vi "SV Software Triggering (Analog Edge).vi"(0 "input signals":waveform(dbl)[](array[waveform]), 1 "restart (F = first call)":bool, 2 "force trigger (F)":bool, 5 "level trigger configuration":T1={"level"=0.0, "slope"=1, "hysteresis"=0.0} {"hysteresis" format="%.2p"; "slope" items=["Falling", "Rising"]; "level" format="%.2p"}, 7 "trigger channel index (0)":i32, 9 "mode (FIFO)":enum16{"First In, First Out", "Last Available"}(ring), 11 "error in (no error)":errorcluster, 12 "pretrigger samples (0)":i32) -> (3 "data timestamp":timestamp, 4 "triggered signals":waveform(dbl)[](array[waveform]), 6 "output ready":bool, 8 "new trigger detected":bool, 15 "error out":errorcluster)   [LabVIEW 2017]
doc: "Implements a software trigger. When the trigger is detected on the trigger channel, all signals are triggered so that the channels stay aligned in time. This function requires that each waveform in <B>input signals</B> has equal <B>dt</B> and <B>Y</B> (length). Returns one triggered set of data per call."
uses:
  <vilib>/addons/_NISVFA/_Shared subVIs/Controls/svc_Analog Level Trigger Configuration.ctl
  <vilib>/addons/_NISVFA/_Shared subVIs/Common/svc_Get Array Subset (Index).vi
  <vilib>/addons/_NISVFA/_Shared subVIs/Common/svc_Check for Waveform Parameter Continuity (no state).vi
  <vilib>/addons/_NISVFA/_Shared subVIs/Common/svc_Coerce Index and Length.vi
  <vilib>/addons/_NISVFA/_Shared subVIs/Common/svc_Get SV Channel Info.vi
  <vilib>/measure/mamon.llb/Trigger Detection for 1 Channel.vi
  <vilib>/addons/_NISVFA/_Shared subVIs/Common/svc_Engineering Units to Unit Label.vi
  <vilib>/addons/_NISVFA/_Shared subVIs/Common/svc_Unit Label to Engineering Units.vi
  <vilib>/measure/NI_MAPro.lvlib
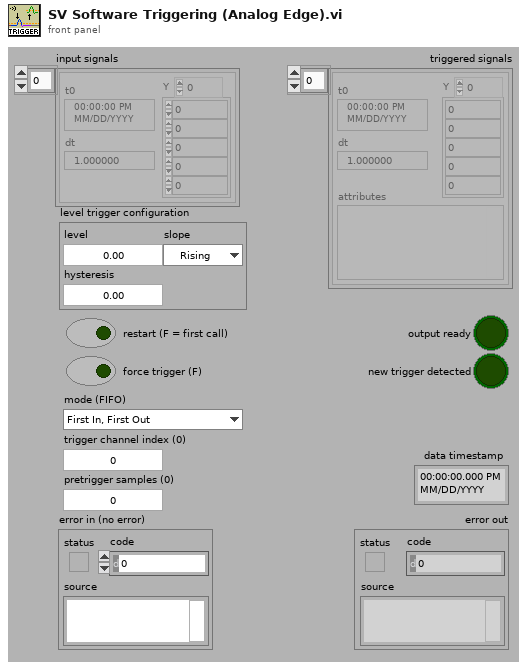
[diagram p1: front panel]
types:
  T1 = typedef "svc_Analog Level Trigger Configuration.ctl" = cluster{"level":dbl, "slope":u16, "hysteresis":dbl}
  T2 = cluster{"dt equal":bool, "array length equal":bool, "number channels change":bool}
  T3 = cluster{"dt":bool, "t0 continuity":bool, "array length":bool, "channel info":bool, "name":bool}
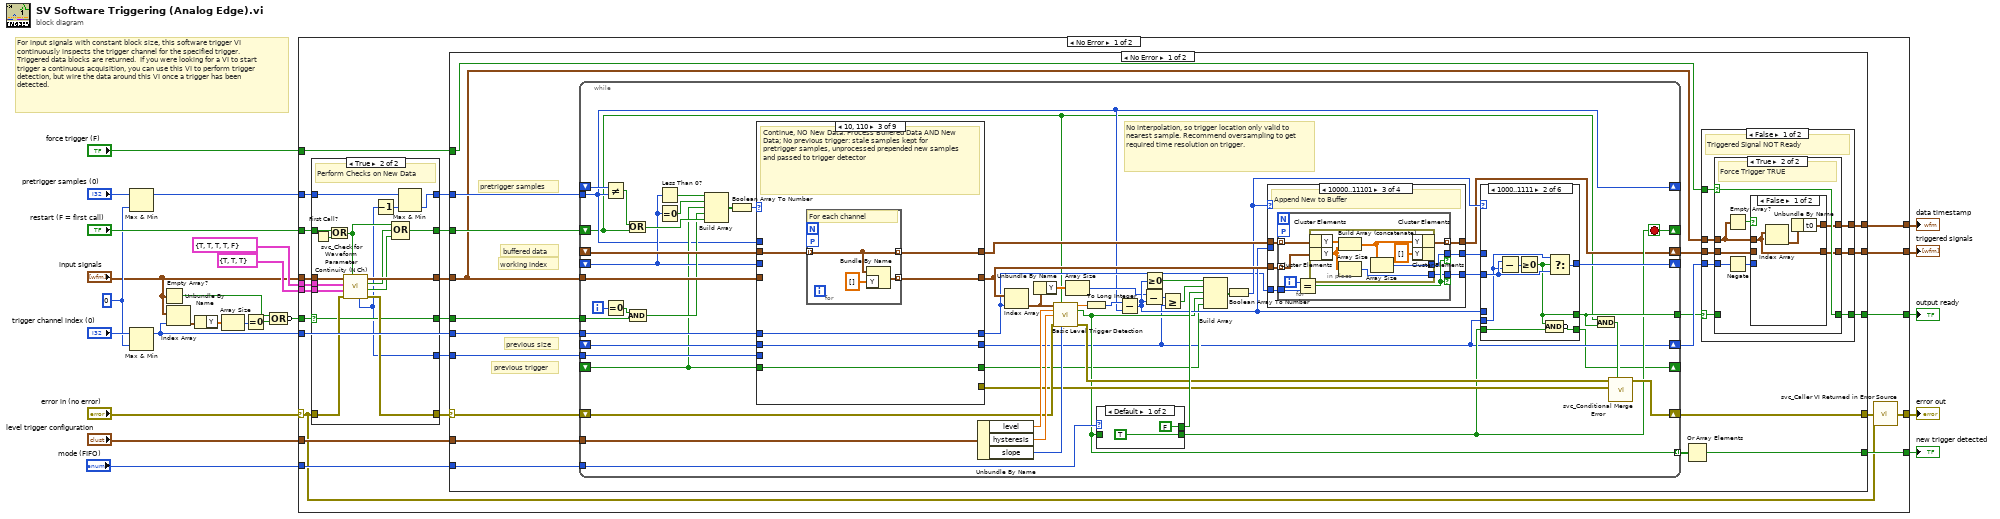
[diagram p0: block diagram]
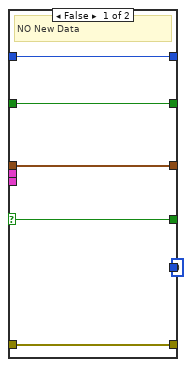
[diagram p2: hidden frame]
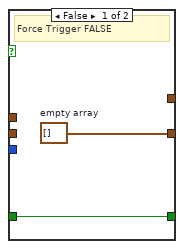
[diagram p3: hidden frame]
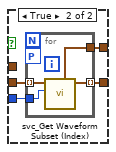
[diagram p4: hidden frame]
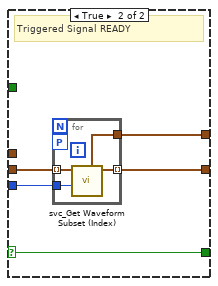
[diagram p5: hidden frame]
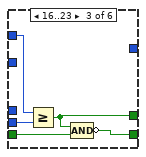
[diagram p7: hidden frame]
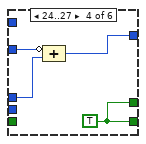
[diagram p8: hidden frame]
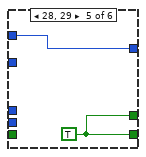
[diagram p9: hidden frame]
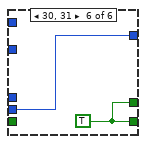
[diagram p10: hidden frame]
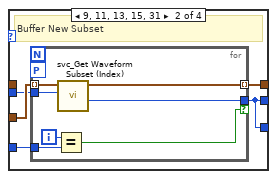
[diagram p12: hidden frame]
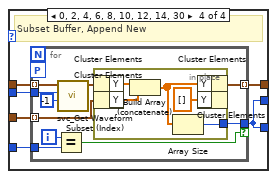
[diagram p13: hidden frame]
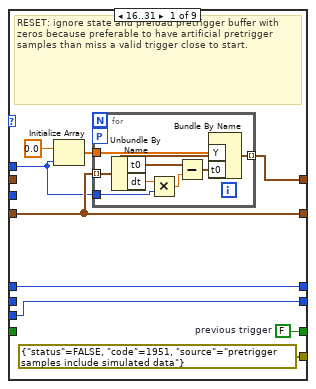
[diagram p14: hidden frame]
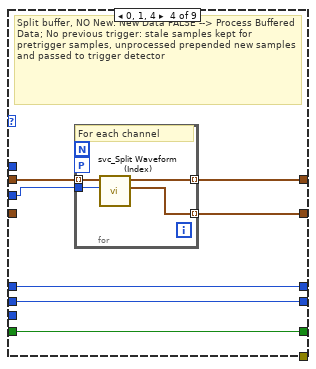
[diagram p16: hidden frame]
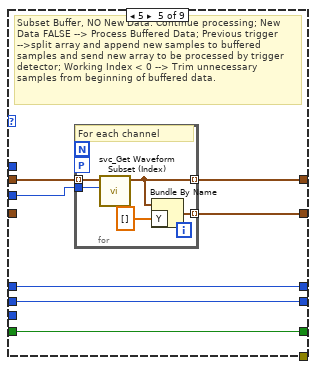
[diagram p17: hidden frame]
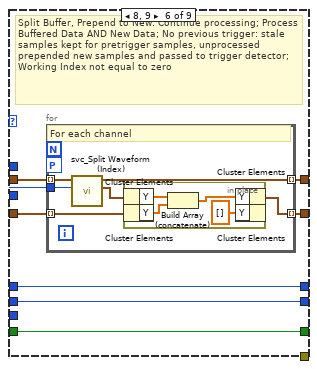
[diagram p18: hidden frame]
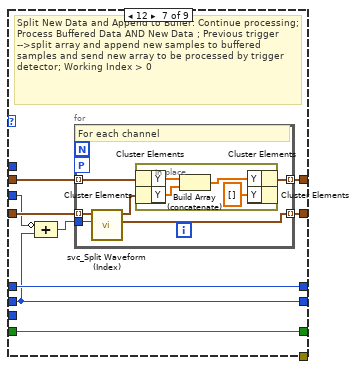
[diagram p19: hidden frame]
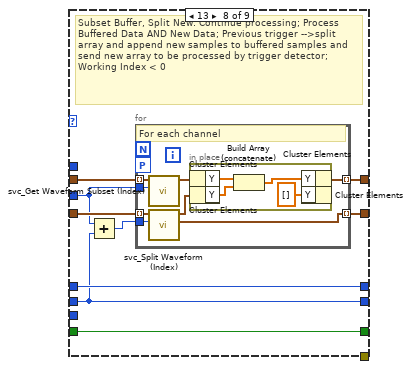
[diagram p20: hidden frame]
diagram:
  w11 = 0 ("y")
  # "For input signals with constant block size, this software trigger VI continuously inspects the trigger channel for the specified trigger. Triggered data blocks are returned.  If you were looking for a VI to start trigger a continuous acquisition, you can use this VI to perform trigger detection, but wire the data around this VI once a trigger has been detected."
  n1 = Max & Min(x="pretrigger samples (0)", y=w11) -> (max(x,y)=w6:i32)  [unwired: 1 out]
  n2 = Max & Min(x="trigger channel index (0)", y=w11) -> (max(x,y)=w13:i32)  [unwired: 1 out]
  n3 = Empty Array?(array="input signals") -> (empty?=w18:bool)
  n4 = Index Array(array="input signals", index=w13) -> (element=w9:waveform(dbl))
  n5 = Unbundle By Name(w9) -> ("Y"=w10:dbl[])
  n6 = Array Size(array=w10) -> (size(s)=w8:i32)
  n7 = Equal To 0?(x=w8) -> (x = 0?=w17:bool)
  n8 = Compound Arithmetic op=OR(w18, w17) -> (invert w4:bool)
  n9 = case shown="No Error" "error in (no error)" {
    selector: "error in (no error)" -> [w26 w380]
    tunnel: "input signals" -> [w42 _]
    tunnel: w13 -> [w47 _]
    tunnel: [w46 _] -> w24
    tunnel: [w45 _] -> w23
    tunnel: [w37 _] -> w22
    tunnel: "level trigger configuration" -> [w44 _]
    tunnel: [w28 w380] -> w20
    tunnel: "restart (F = first call)" -> [w43 _]
    tunnel: T2 {"dt equal"=TRUE, "array length equal"=TRUE, "number channels change"=TRUE} ("checks for multichannel parameters") -> [w40 _]
    tunnel: T3 {"dt"=TRUE, "t0 continuity"=TRUE, "array length"=TRUE, "channel info"=TRUE, "name"=FALSE} ("checks for channel parameter change") -> [w39 _]
    tunnel: "force trigger (F)" -> [w35 _]
    tunnel: w6 -> [w34 _]
    tunnel: w4 -> [w32 _]
    tunnel: "mode (FIFO)" -> [w29 _]
    tunnel: [w25 _] -> w1
    frame No Error {
      n10 = case shown="True" w32 {
        selector: w32 -> [w48 w55]
        tunnel: w43 -> [w50 w70]
        tunnel: w42 -> [w53 w68]
        tunnel: [w53 w67] -> w41
        tunnel: w26 -> [w52 w66]
        tunnel: w40 -> [_ w65]
        tunnel: w39 -> [_ w64]
        tunnel: [w50 w60] -> w38
        tunnel: [w52 w59] -> w36
        tunnel: w34 -> [w51 w57]
        tunnel: [w51 w56] -> w33
        tunnel: [0 ("array length") w54] -> w31
        tunnel: [w48 w55] -> w30
        frame False {
          # "NO New Data"
        }
        frame True {
          # "Perform Checks on New Data"
          n11 = First Call?() -> (First Call?: T/F=w69:bool)
          n12 = Or(x=w70, y=w69) -> (x .or. y?=w61:bool)
          n13 = call <vilib>:"svc_Check for Waveform Parameter Continuity (N Ch).vi"("restart averaging (F)"=w61, "error in (no error)"=w66, "checks for multichannel parameters"=w65, "checks for channel parameter change"=w64, "scaled signal(s)"=w68) -> ("error out"=w59:errorcluster, "multichannel parameter changed"=w62:bool, "waveform parameter changed"=w63:bool, "dup scaled signal(s)"=w67:waveform(dbl)[], "array length"=w54:i32)  [unwired: 2 out]
          n14 = Decrement(x=w54) -> (x-1=w58:i32)
          n15 = Compound Arithmetic op=OR(w61, w63, w62) -> (w60:bool)
          n16 = Max & Min(x=w57, y=w58) -> (min(x,y)=w56:i32)  [unwired: 1 out]
        }
      }
      n17 = case shown="No Error" w36 {
        selector: w36 -> [w84 w379]
        tunnel: w33 -> [w89 _]
        tunnel: w47 -> [w88 _]
        tunnel: [w76 _] -> w46
        tunnel: [w73 _] -> w45
        tunnel: w44 -> [w87 _]
        tunnel: [w72 w379] -> w27
        tunnel: w31 -> [w86 _]
        tunnel: w41 -> [w77 _]
        tunnel: w38 -> [w85 _]
        tunnel: [w81 _] -> w37
        tunnel: w35 -> [w78 _]
        tunnel: w30 -> [w75 _]
        tunnel: w29 -> [w74 _]
        tunnel: [w71 _] -> w25
        frame No Error {
          # "pretrigger samples"
          # "previous size"
          # "previous trigger"
          # "working index"
          # "buffered data"
          n18 = while {
            shift-right: [w131] -> w83
            shift-left: _ -> [w162]
            tunnel: w77 -> [w161]
            shift-right: [w128] -> _
            shift-left: _ -> [w136]
            tunnel: w89 -> [w130]
            tunnel: w88 -> [w160]
            tunnel: [w142] -> w80
            shift-right: [w132] -> w82
            shift-left: _ -> [w159]
            tunnel: w87 -> [w180]
            tunnel: w86 -> [w158]
            shift-right: [w146] -> w72
            shift-left: w84 -> [w179]
            shift-right: [w143] -> _
            shift-left: _ -> [w156]
            tunnel: [w137] -> w79 mode=indexing
            shift-right: [w130] -> _
            shift-left: _ -> [w178]
            tunnel: w75 -> [w173]
            tunnel: w74 -> [w155]
            shift-right: [w135] -> _
            shift-left: w85 -> [w129]
            i -> [w175]
            stop <- w135 stop-if-true
            # "No interpolation, so trigger location only valid to nearest sample. Recommend oversampling to get required time resolution on trigger."
            n19 = Not Equal?(x=w178, y=w130) -> (x != y?=w177:bool)
            n20 = Equal To 0?(x=w175) -> (x = 0?=w174:bool)
            n21 = Or(x=w177, y=w129) -> (x .or. y?=w167:bool)
            n22 = And(x=w174, y=w173) -> (x .and. y?=w157:bool)
            n23 = Less Than 0?(x=w156) -> (x < 0?=w165:bool)
            n24 = Equal To 0?(x=w156) -> (x = 0?=w166:bool)
            n25 = Build Array(w165, w166, w136, w157, w167) -> (w164:bool[])
            n26 = Boolean Array To Number(Boolean array=w164) -> (number=w163:u32)
            n27 = case shown="10, 110" w163 {
              tunnel: w161 -> [w261 w278 _ _ _ w315 w334 w354 w372]
              tunnel: w160 -> [w265 w276 w283 w293 w304 w317 w337 w356 w370]
              tunnel: [w260 w275 w284 w294 w305 w318 w330 w349 w373] -> w132
              tunnel: w162 -> [_ w277 w282 w292 w303 w316 w335 w353 w371]
              tunnel: [w261 w278 w281 w291 w302 w314 w332 w351 w372] -> w147
              tunnel: w159 -> [_ w275 w284 w294 w305 w318 w330 w349 w373]
              tunnel: [w262 w277 w280 w290 w300 w313 w333 w352 w371] -> w148
              tunnel: [w265 w276 w283 w293 w304 w317 w337 w356 w370] -> w138
              tunnel: w130 -> [w259 _ _ _ _ _ _ _ _]
              tunnel: w158 -> [w260 _ _ _ _ _ _ _ _]
              tunnel: w156 -> [_ _ _ w289 w301 w312 w331 w350 _]
              tunnel: [errorcluster {"status"=FALSE, "code"=1951, "source"="pretrigger samples include simulated data"} ("error in 2 (no error)") _ _ _ _ _ _ _ _] -> w149
              tunnel: w136 -> [_ w274 w279 w288 w299 w311 w329 w348 w369]
              tunnel: [w257 w274 w279 w288 w299 w311 w329 w348 w369] -> w133
              frame 16..31 {
                w257 = FALSE  # previous trigger
                # "RESET: ignore state and preload pretrigger buffer with zeros because preferable to have artificial pretrigger samples than miss a valid trigger close to start."
                n28 = Initialize Array(0.0 ("element"), w259) -> (w263:dbl[])
                n29 = for {
                  tunnel: w261 -> [w272] mode=indexing
                  tunnel: w263 -> [w266]
                  tunnel: [w273] -> w262 mode=indexing
                  tunnel: w259 -> [w270]
                  workers-P: _ -> [_]
                  n30 = Unbundle By Name(w272) -> ("t0"=w269:timestamp, "dt"=w271:dbl)
                  n31 = Multiply(x=w271, y=w270) -> (x*y=w268:dbl)
                  n32 = Subtract(x=w269, y=w268) -> (x-y=w267:timestamp)
                  n33 = Bundle By Name(cluster=w272, "Y"=w266, "t0"=w267) -> (w273:waveform(dbl))
                }
              }
              frame 10, 14 {
                # "Continue with pass through: Process Buffered Data AND New Data; Working Index = 0 (all buffered samples have been inspected)"
              }
              frame 2, 6 {
                # "Continue, NO New Data: Process Buffered Data AND New Data; No previous trigger: stale samples kept for pretrigger samples, unprocessed prepended new samples and passed to trigger detector"
                n34 = for {
                  tunnel: [w286] -> w280 mode=indexing
                  tunnel: w282 -> [w286] mode=indexing
                  tunnel: [w285] -> w281 mode=indexing
                  workers-P: _ -> [_]
                  # "For each channel"
                  n35 = Bundle By Name(cluster=w286, "Y"=dbl[] []) -> (w285:waveform(dbl))
                }
              }
              frame 0, 1, 4 {
                # "Split buffer, NO New: New Data FALSE --> Process Buffered Data; No previous trigger: stale samples kept for pretrigger samples, unprocessed prepended new samples and passed to trigger detector"
                n36 = for {
                  tunnel: w292 -> [w298] mode=indexing
                  tunnel: w289 -> [w297]
                  tunnel: [w296] -> w290 mode=indexing
                  tunnel: [w295] -> w291 mode=indexing
                  workers-P: _ -> [_]
                  # "For each channel"
                  n37 = call <vilib>:"svc_Split Waveform (Index).vi"("index"=w297, "waveform in"=w298) -> ("second waveform out"=w295:waveform(dbl), "first waveform out"=w296:waveform(dbl))  [unwired: 7 in, 1 out]
                }
              }
              frame 5 {
                # "Subset Buffer, NO New Data: Continue processing; New Data FALSE --> Process Buffered Data; Previous trigger -->split array and append new samples to buffered samples and send new array to be processed by trigger detector; Working Index < 0 --> Trim unnecessary samples from beginning of buffered data."
                n38 = for {
                  tunnel: w303 -> [w310] mode=indexing
                  tunnel: [w308] -> w300 mode=indexing
                  tunnel: w301 -> [w309]
                  workers-P: _ -> [_]
                  tunnel: [w306] -> w302 mode=indexing
                  # "For each channel"
                  n39 = call <vilib>:"svc_Get Waveform Subset (Index).vi"("start index (0)"=w309, "waveform in"=w310) -> ("waveform subset"=w308:waveform(dbl))  [unwired: 4 in, 5 out]
                  n40 = Bundle By Name(cluster=w308, "Y"=dbl[] []) -> (w306:waveform(dbl))
                }
              }
              frame 8, 9 {
                # "Split Buffer, Prepend to New: Continue processing; Process Buffered Data AND New Data; No previous trigger: stale samples kept for pretrigger samples, unprocessed prepended new samples and passed to trigger detector; Working Index not equal to zero"
                n41 = for {
                  tunnel: w316 -> [w324] mode=indexing
                  tunnel: w315 -> [w320] mode=indexing
                  tunnel: w312 -> [w323]
                  tunnel: [w322] -> w313 mode=indexing
                  tunnel: [w319] -> w314 mode=indexing
                  workers-P: _ -> [_]
                  # "For each channel"
                  n42 = call <vilib>:"svc_Split Waveform (Index).vi"("index"=w323, "waveform in"=w324) -> ("second waveform out"=w321:waveform(dbl), "first waveform out"=w322:waveform(dbl))  [unwired: 7 in, 1 out]
                  n43 = in-place {
                    n44 = in-place-cluster #1(w321) -> ("Y"=w328:dbl[])
                    n45 = in-place-cluster #2(w320) -> ("Y"=w327:dbl[])
                    n46 = Build Array (concatenate)(w328, w327) -> (w326:dbl[])
                    n47 = in-place-cluster #1("Y"=w326) -> (w319:waveform(dbl))
                    n48 = in-place-cluster #2("Y"=dbl[] []) -> ()  [unwired: 1 out]
                  }
                }
              }
              frame 12 {
                # "Split New Data and Append to Buffer: Continue processing; Process Buffered Data AND New Data ; Previous trigger -->split array and append new samples to buffered samples and send new array to be processed by trigger detector; Working Index > 0"
                n49 = Compound Arithmetic op=ADD(invert w331, w330) -> (w336:i32)
                n50 = for {
                  tunnel: w335 -> [w340] mode=indexing
                  tunnel: [w341] -> w332 mode=indexing
                  tunnel: w334 -> [w343] mode=indexing
                  tunnel: [w338] -> w333 mode=indexing
                  tunnel: w336 -> [w342]
                  workers-P: _ -> [_]
                  # "For each channel"
                  n51 = call <vilib>:"svc_Split Waveform (Index).vi"("index"=w342, "waveform in"=w343) -> ("second waveform out"=w341:waveform(dbl), "first waveform out"=w339:waveform(dbl))  [unwired: 7 in, 1 out]
                  n52 = in-place {
                    n53 = in-place-cluster #3(w340) -> ("Y"=w347:dbl[])
                    n54 = in-place-cluster #4(w339) -> ("Y"=w346:dbl[])
                    n55 = Build Array (concatenate)(w347, w346) -> (w345:dbl[])
                    n56 = in-place-cluster #3("Y"=w345) -> (w338:waveform(dbl))
                    n57 = in-place-cluster #4("Y"=dbl[] []) -> ()  [unwired: 1 out]
                  }
                }
              }
              frame 13 {
                # "Subset Buffer, Split New: Continue processing; Process Buffered Data AND New Data; Previous trigger -->split array and append new samples to buffered samples and send new array to be processed by trigger detector; Working Index < 0"
                n58 = Add(x=w350, y=w349) -> (x+y=w355:i32)
                n59 = for {
                  tunnel: w353 -> [w362] mode=indexing
                  tunnel: [w363] -> w351 mode=indexing
                  tunnel: w354 -> [w364] mode=indexing
                  tunnel: [w357] -> w352 mode=indexing
                  tunnel: w350 -> [w361]
                  tunnel: w355 -> [w360]
                  workers-P: _ -> [_]
                  # "For each channel"
                  n60 = call <vilib>:"svc_Get Waveform Subset (Index).vi"("start index (0)"=w361, "waveform in"=w362) -> ("waveform subset"=w359:waveform(dbl))  [unwired: 4 in, 5 out]
                  n61 = call <vilib>:"svc_Split Waveform (Index).vi"("index"=w360, "waveform in"=w364) -> ("second waveform out"=w363:waveform(dbl), "first waveform out"=w358:waveform(dbl))  [unwired: 7 in, 1 out]
                  n62 = in-place {
                    n63 = in-place-cluster #5(w359) -> ("Y"=w368:dbl[])
                    n64 = in-place-cluster #6(w358) -> ("Y"=w367:dbl[])
                    n65 = Build Array (concatenate)(w368, w367) -> (w366:dbl[])
                    n66 = in-place-cluster #5("Y"=w366) -> (w357:waveform(dbl))
                    n67 = in-place-cluster #6("Y"=dbl[] []) -> ()  [unwired: 1 out]
                  }
                }
              }
              frame 3, 7, 11, 15, Default {
                # "Unused Cases (because working index cannot be both =0 AND <0)\nDefault case --> You should never be here!"
              }
            }
            n68 = Unbundle By Name(w180) -> ("level"=w182:dbl, "hysteresis"=w181:dbl, "slope"=w172:u16)
            n69 = Index Array(array=w147, index=w138) -> (element=w170:waveform(dbl))
            n70 = Unbundle By Name(w170) -> ("Y"=w171:dbl[])
            n71 = call-poly <vilib>:"Basic Level Trigger Detection.vi"("signal in"=w170, "reset"=w129, "level"=w182, "hysteresis"=w181, "error in (no error)"=w179, "trigger slope"=w172) -> ("trigger location"=w176:dbl, "trigger detected?"=w137:bool, "error out"=w141:errorcluster)  [unwired: 7 in]
            n72 = Array Size(array=w171) -> (size(s)=w134:i32)
            n73 = To Long Integer(number=w176) -> (32bit integer=w168:i32)
            n74 = case shown="Default" w155 {
              tunnel: [TRUE w377] -> w135
              tunnel: w137 -> [_ w378]
              tunnel: [FALSE TRUE] -> w153
              frame Default {
              }
              frame "Last Available" {
                n75 = Not(x=w378) -> (.not. x?=w377:bool)
              }
            }
            n76 = Subtract(x=w168, y=w130) -> (x-y=w139:i32)
            n77 = Subtract(x=w134, y=w139) -> (x-y=w169:i32)
            n78 = Greater Or Equal To 0?(x=w139) -> (x >= 0?=w151:bool)
            n79 = Greater Or Equal?(x=w169, y=w132) -> (x >= y?=w152:bool)
            n80 = Build Array(w151, w152, w153, w137, w133) -> (w154:bool[])
            n81 = Boolean Array To Number(Boolean array=w154) -> (number=w140:u32)
            n82 = case shown="10000..11101" w140 {
              tunnel: w147 -> [w203 w208 w220 w240]
              tunnel: w139 -> [_ w205 _ w238]
              tunnel: w148 -> [_ _ w221 w241]
              tunnel: w138 -> [_ w206 w218 w237]
              tunnel: [w203 w207 w219 w239] -> w131
              tunnel: [_ w204 w216 w236] -> w145
              tunnel: [_ w204 w217 w236] -> w144
              frame 1, 3, 5, 7, Default {
                # "NO Triggers, Buffer New:"
              }
              frame 9, 11, 13, 15, 31 {
                # "Buffer New Subset"
                n83 = for {
                  tunnel: w208 -> [w215] mode=indexing
                  tunnel: w205 -> [w214]
                  tunnel: [w213] -> w207 mode=indexing
                  tunnel: [w212] -> w204 if=w209
                  tunnel: w206 -> [w211]
                  workers-P: _ -> [_]
                  i -> [w210]
                  n84 = Equal?(x=w210, y=w211) -> (x = y?=w209:bool)
                  n85 = call <vilib>:"svc_Get Waveform Subset (Index).vi"("start index (0)"=w214, "waveform in"=w215) -> ("actual length"=w212:i32, "waveform subset"=w213:waveform(dbl))  [unwired: 4 in, 4 out]
                }
              }
              frame 16..29 {
                # "Append New to Buffer"
                n86 = for {
                  tunnel: w220 -> [w225] mode=indexing
                  tunnel: [w224] -> w219 mode=indexing
                  tunnel: w221 -> [w226] mode=indexing
                  tunnel: w218 -> [w228]
                  tunnel: [w222] -> w216 if=w227
                  tunnel: [w223] -> w217 if=w227
                  workers-P: _ -> [_]
                  i -> [w229]
                  n87 = Equal?(x=w229, y=w228) -> (x = y?=w227:bool)
                  n88 = in-place {
                    in-place-border: [w231] -> w223
                    in-place-border: [w230] -> w222
                    n89 = in-place-cluster #7(w226) -> ("Y"=w235:dbl[])
                    n90 = in-place-cluster #8(w225) -> ("Y"=w233:dbl[])
                    n91 = Build Array (concatenate)(w235, w233) -> (w232:dbl[])
                    n92 = Array Size(array=w233) -> (size(s)=w230:i32)
                    n93 = Array Size(array=w232) -> (size(s)=w231:i32)
                    n94 = in-place-cluster #7("Y"=w232) -> (w224:waveform(dbl))
                    n95 = in-place-cluster #8("Y"=dbl[] []) -> ()  [unwired: 1 out]
                  }
                }
              }
              frame 0, 2, 4, 6, 8, 10, 12, 14, 30 {
                # "Subset Buffer, Append New"
                n96 = for {
                  tunnel: w240 -> [w243] mode=indexing
                  tunnel: [w245] -> w239 mode=indexing
                  tunnel: w241 -> [w251] mode=indexing
                  tunnel: w238 -> [w250]
                  tunnel: w237 -> [w247]
                  tunnel: [w242] -> w236 if=w246
                  workers-P: _ -> [_]
                  i -> [w248]
                  n97 = Equal?(x=w248, y=w247) -> (x = y?=w246:bool)
                  n98 = call <vilib>:"svc_Get Waveform Subset (Index).vi"("length (-1 = all)"=-1 ("length"), "start index (0)"=w250, "waveform in"=w251) -> ("waveform subset"=w244:waveform(dbl))  [unwired: 3 in, 5 out]
                  n99 = in-place {
                    in-place-border: [w252] -> w242
                    n100 = in-place-cluster #9(w244) -> ("Y"=w256:dbl[])
                    n101 = in-place-cluster #10(w243) -> ("Y"=w254:dbl[])
                    n102 = Build Array (concatenate)(w256, w254) -> (w253:dbl[])
                    n103 = Array Size(array=w253) -> (size(s)=w252:i32)
                    n104 = in-place-cluster #9("Y"=w253) -> (w245:waveform(dbl))
                    n105 = in-place-cluster #10("Y"=dbl[] []) -> ()  [unwired: 1 out]
                  }
                }
              }
            }
            n106 = case shown="1000..1111" w140 {
              tunnel: w145 -> [_ w188 _ w198 _ _]
              tunnel: w132 -> [_ w183 w194 _ _ w202]
              tunnel: [_ w187 w191 w196 w200 w201] -> w142
              tunnel: w135 -> [_ w186 w190 _ _ _]
              tunnel: [_ w185 _ w197 w199 w202] -> w143
              tunnel: [_ w184 w193 w196 w200 w201] -> w128
              tunnel: w144 -> [_ _ w192 _ w199 _]
              tunnel: w139 -> [_ _ _ w195 _ _]
              frame 0..7, Default {
              }
              frame 8..15 {
                n107 = Subtract(x=w188, y=w183) -> (x-y=w189:i32)
                n108 = Greater Or Equal To 0?(x=w189) -> (x >= 0?=w187:bool)
                n109 = Compound Arithmetic op=AND(w187, w186) -> (invert w184:bool)
                n110 = Select(t=w183, s=w187, f=w188) -> (s? t:f=w185:i32)
              }
              frame 16..23 {
                n111 = Greater Or Equal?(x=w192, y=w194) -> (x >= y?=w191:bool)
                n112 = Compound Arithmetic op=AND(w191, w190) -> (invert w193:bool)
              }
              frame 24..27 {
                w196 = TRUE
                n113 = Compound Arithmetic op=ADD(invert w198, w195) -> (w197:i32)
              }
              frame 28, 29 {
                w200 = TRUE
              }
              frame 30, 31 {
                w201 = TRUE
              }
            }
            n114 = And(x=w129, y=w142) -> (x .and. y?=w150:bool)
            n115 = call <vilib>:"svc_Conditional Merge Error.vi"("merge"=w150, "new error"=w149, "error in (no error)"=w141) -> ("error out"=w146:errorcluster)  [unwired: 8 in]
          }
          n116 = Or Array Elements(Boolean array=w79) -> (logical OR=w73:bool)
          n117 = case shown="False" w80 {
            selector: w80 -> [w93 w120]
            tunnel: w83 -> [w92 w123]
            tunnel: w82 -> [w91 w122]
            tunnel: [w97 w121] -> w81
            tunnel: w78 -> [w96 _]
            tunnel: w77 -> [w95 _]
            tunnel: [w94 w120] -> w76
            tunnel: [w90 w119] -> w71
            frame False {
              # "Triggered Signal NOT Ready"
              n118 = case shown="True" w96 {
                selector: w96 -> [_ w107]
                tunnel: [w99 w105] -> w97
                tunnel: w95 -> [_ w104]
                tunnel: [w98 w107] -> w94
                tunnel: w93 -> [w98 _]
                tunnel: w92 -> [_ w103]
                tunnel: w91 -> [_ w102]
                tunnel: [_ w100] -> w90
                frame False {
                  w99 = waveform(dbl)[] []  # empty array
                  # "Force Trigger FALSE"
                }
                frame True {
                  # "Force Trigger TRUE"
                  n119 = Empty Array?(array=w104) -> (empty?=w106:bool)
                  n120 = Negate(x=w102) -> (-x=w101:i32)
                  n121 = case shown="False" w106 {
                    tunnel: [w108 w113] -> w105
                    tunnel: w104 -> [w108 _]
                    tunnel: w103 -> [_ w114]
                    tunnel: w101 -> [_ w112]
                    tunnel: [w109 w111] -> w100
                    frame False {
                      n122 = Index Array(array=w108) -> (element=w110:waveform(dbl))  [unwired: 1 in]
                      n123 = Unbundle By Name(w110) -> ("t0"=w109:timestamp)
                    }
                    frame True {
                      n124 = for {
                        tunnel: w114 -> [w118] mode=indexing
                        tunnel: [w117] -> w113 mode=indexing
                        workers-P: _ -> [_]
                        tunnel: w112 -> [w116]
                        tunnel: [w115] -> w111
                        n125 = call <vilib>:"svc_Get Waveform Subset (Index).vi"("start index (0)"=w116, "waveform in"=w118) -> ("waveform subset"=w117:waveform(dbl), "subset timestamp"=w115:timestamp)  [unwired: 4 in, 4 out]
                      }
                    }
                  }
                }
              }
            }
            frame True {
              # "Triggered Signal READY"
              n126 = for {
                tunnel: w123 -> [w127] mode=indexing
                tunnel: w122 -> [w126]
                tunnel: [w125] -> w121 mode=indexing
                workers-P: _ -> [_]
                tunnel: [w124] -> w119
                n127 = call <vilib>:"svc_Get Waveform Subset (Index).vi"("length (-1 = all)"=w126, "waveform in"=w127) -> ("waveform subset"=w125:waveform(dbl), "subset timestamp"=w124:timestamp)  [unwired: 4 in, 4 out]
              }
            }
          }
        }
        frame Error {
        }
      }
      n128 = call <vilib>:"svc_Caller VI Returned in Error Source.vi"("warning input to caller"=w26, "error in (no error)"=w27) -> ("error out"=w28:errorcluster)  [unwired: 3 in]
    }
    frame Error {
    }
  }
  "new trigger detected" <- w23
  "output ready" <- w24
  "triggered signals" <- w22
  "error out" <- w20
  "data timestamp" <- w1
